vi "Main.vi"() -> ()   [LabVIEW 2019, in "Streamer_server.lvlib" / "Streamer_server.lvclass"]
uses:
  Streamer_server.lvclass
  typeDefs/Server State Data.ctl
  Streamer_server.lvclass/Streamer_server.ctl
panel:
  out "Listening Port":i32
  in  "Stop":bool
  in  "Server Address":string="localhost:50051"
  in  "Server Certificate File (.crt)":path
  in  "Server Key File (.key)":path
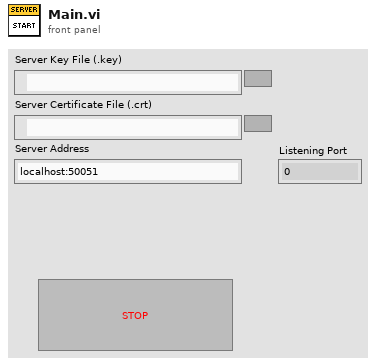
[diagram p1: front panel]
types:
  T1 = typedef "Streamer_server.lvlib/Streamer_server.lvclass/Server State Data.ctl" = cluster{"Data":string}
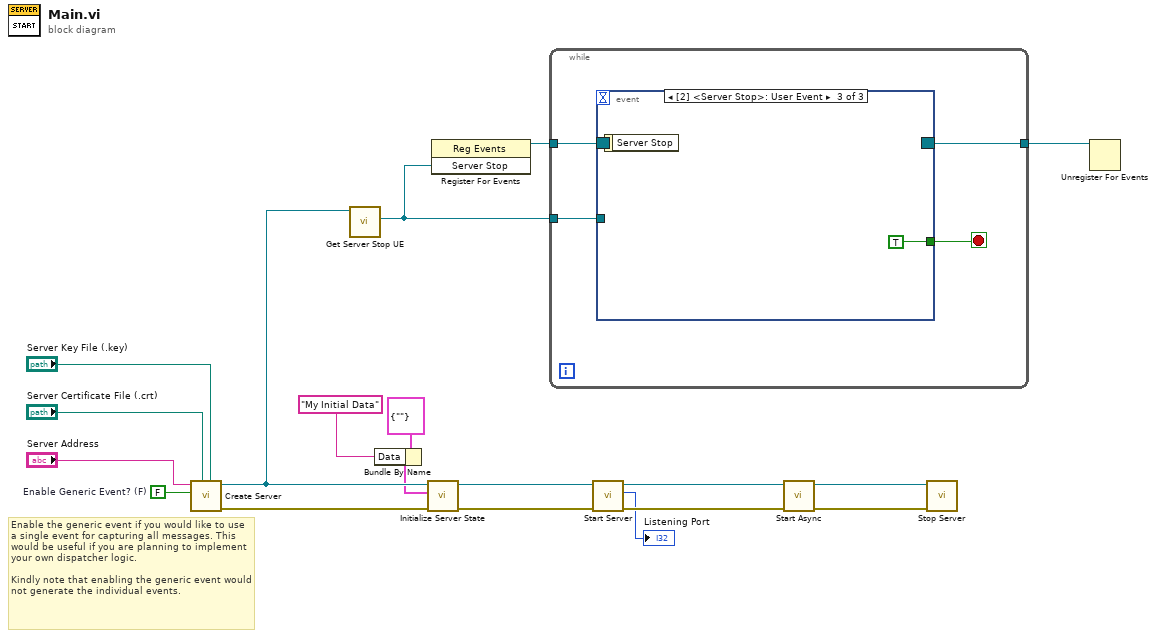
[diagram p0: block diagram]
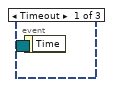
[diagram p2: hidden frame]
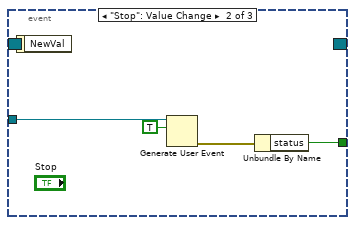
[diagram p3: hidden frame]
diagram:
  w1 = FALSE  # Enable Generic Event? (F)
  # "Enable the generic event if you would like to use a single event for capturing all messages. This would be useful if you are planning to implement your own dispatcher logic. \n\nKindly note that enabling the generic event would not generate the individual events."
  n1 = call "Create Server.vi"("Server Key File (.key)"="Server Key File (.key)", "Server Certificate File (.crt)"="Server Certificate File (.crt)", "Enable Generic Event? (F)"=w1, "Server Address"="Server Address") -> ("error out"=w9:errorcluster, "gRPC Server out"=w6:refnum<class "Streamer_server.lvclass">)  [unwired: 6 in]
  n2 = call "Get Server Stop UE.vi"("OOP Server in"=w6) -> ("Server Stop"=w10:refnum<user-event>)  [unwired: 9 in, 1 out]
  n3 = Bundle By Name(cluster=T1 {"Data"=""} ("Initial State"), "Data"="My Initial Data") -> (w4:T1)
  n4 = call "Initialize Server State.vi"("error in (no error)"=w9, "Initial State"=w4, "gRPC Server in"=w6) -> ("error out"=w8:errorcluster, "gRPC Server out"=w7:refnum<class "Streamer_server.lvclass">)  [unwired: 7 in]
  n5 = register-events(w10) -> (reference out=w12:refnum<event-registration>)  [unwired: 2 in, 1 out]
  n6 = while {
    tunnel: w10 -> [w23]
    tunnel: w12 -> [w22]
    tunnel: [w20] -> w11
    stop <- w21 stop-if-true
    n7 = event shown="[2] <Server Stop>: User Event" {
      selector: w22 -> [_ _ _]
      dyn-events: [_ _ _] -> w20
      timeout: _ -> [_ _ _]
      tunnel: w23 -> [_ w27 _]
      tunnel: [_ w24 TRUE] -> w21
      event Timeout {
        n8 = event-data() -> ()  [unwired: 1 in, 1 out]
      }
      event "Stop": Value Change {
        n9 = event-data() -> ()  [unwired: 1 in, 1 out]
        n10 = Generate User Event(user event=w27, event data cluster=TRUE ("event data")) -> (error out=w25:errorcluster)  [unwired: 2 in, 1 out]
        n11 = Unbundle By Name(w25) -> ("status"=w24:bool)
      }
      event User Event {
        n12 = event-data() -> ()  [unwired: 1 in, 1 out]
      }
    }
  }
  n13 = call "Start Server.vi"("error in (no error)"=w8, "gRPC Server in"=w7) -> ("error out"=w19:errorcluster, "Listening Port"=→"Listening Port":i32, "gRPC Server out"=w18:refnum<class "Streamer_server.lvclass">)  [unwired: 7 in]
  n14 = call "Start Async.vi"("error in (no error)"=w19, "gRPC Server in"=w18) -> ("error out"=w17:errorcluster, "gRPC Server out"=w16:refnum<class "Streamer_server.lvclass">)  [unwired: 8 in]
  n15 = call "Stop Server.vi"("error in (no error)"=w17, "gRPC Server in"=w16) -> ()  [unwired: 9 in, 1 out]
  n16 = Unregister For Events(event registration refnum=w11) -> ()  [unwired: 1 in, 1 out]
